vi "CFU_6p1_006.vi"() -> ()   [LabVIEW 2016]
uses:
  <vilib>/express/express arith-compare/Formula/XNode/ExpressFormulaBlockNode.xnode
panel:
  out "d = minimum diameter (mm)":dbl
  in  "Sigma =Design stress (MPa)":dbl
  in  "F=Force (N)":dbl
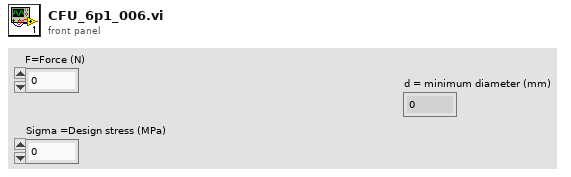
[diagram p1: front panel]
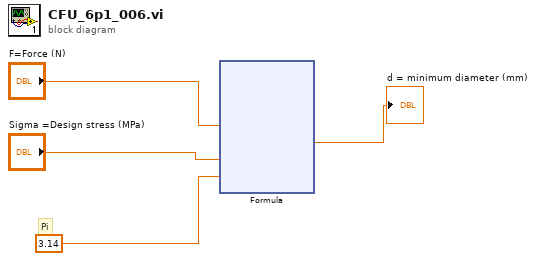
[diagram p0: block diagram]
diagram:
  # "Pi"
  n1 = xnode "Formula"("F"="F=Force (N)", "Sigma"="Sigma =Design stress (MPa)", "pi"=3.14) -> ("Result"=→"d = minimum diameter (mm)":dbl)  [unwired: 1 in, 1 out]
